vi "item select select all.vi"(8 "error in (no error)":errorcluster, 11 "Listbox or Tree":refnum<vi>) -> (0 "error out":errorcluster, 3 "Ref":refnum<vi>)   [LabVIEW 2020, in "UI_ItemSelect.lvlib"]
uses:
  UI_ItemSelect.lvlib
  SubVIs/item select action.ctl
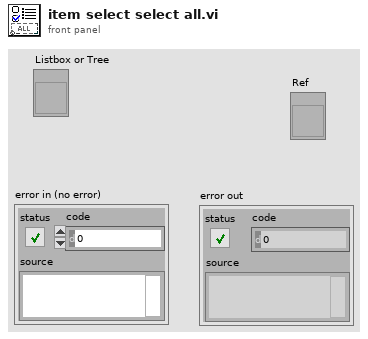
[diagram p1: front panel]
types:
  T1 = typedef "UI_ItemSelect.lvlib/item select action.ctl" = enum16{"init", "read", "write states", "write locks", "mouse down", "delete", "select all", "select none", "invert selection"}
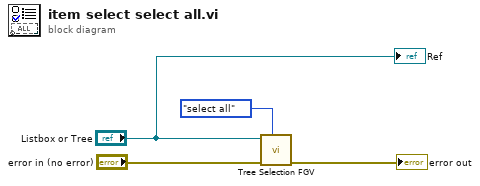
[diagram p0: block diagram]
diagram:
  n1 = call "Tree Selection FGV.vi"("Action"=item_select_action."select all", "error in (no error)"="error in (no error)", "Listbox or Tree"="Listbox or Tree") -> ("error out"=→"error out":errorcluster)  [unwired: 7 in, 1 out]
  "Ref" <- "Listbox or Tree"
